vi "uut_status.vi"(8 "error in (no error)":errorcluster, 11 "status":bool) -> (0 "error out":errorcluster)   [LabVIEW 2019]
panel:
  out "String":string
  out "status":string
  # "UUT Status"
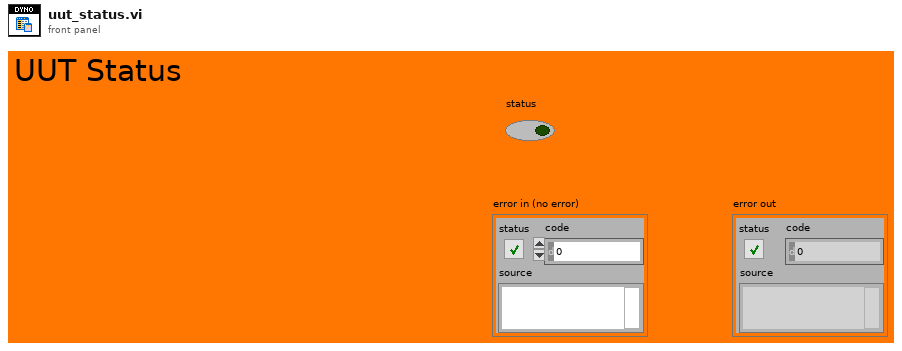
[diagram p1: front panel]
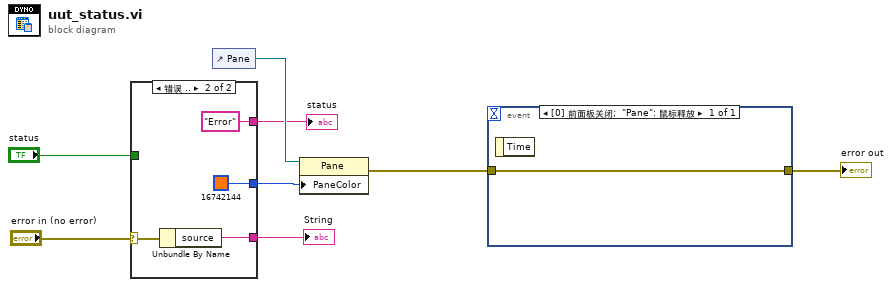
[diagram p0: block diagram]
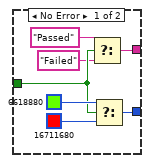
[diagram p2: hidden frame]
diagram:
  n1 = case shown="错误 .." "error in (no error)" {
    selector: "error in (no error)" -> [_ w17]
    tunnel: "status" -> [w12 _]
    tunnel: [w13 u32 16742144] -> w3
    tunnel: [w11 "Error"] -> w2
    tunnel: [_ w16] -> w1
    frame No Error {
      n2 = Select(t="Passed" ("status"), s=w12, f="Failed" ("status")) -> (s? t:f=w11:string)
      n3 = Select(t=u32 6618880, s=w12, f=u32 16711680) -> (s? t:f=w13:u32)
    }
    frame Error {
      n4 = Unbundle By Name(w17) -> ("source"=w16:string)
    }
  }
  "status" <- w2
  "String" <- w1
  n5 = control-ref of="Pane"() -> (w7:refnum<vi>)
  n6 = property class="Pane"(reference=w7, "PaneColor"=w3) -> (error out=w6:errorcluster)  [unwired: 1 in, 1 out]
  n7 = event shown="[0] 前面板关闭;  \"Pane\": 鼠标释放" {
    selector: _ -> [_]
    dyn-events: _ -> [_]
    timeout: _ -> [_]
    tunnel: [w20] -> w8
    tunnel: w6 -> [w20]
    event Panel Close; Mouse Up {
      n8 = event-data() -> ()  [unwired: 1 in, 1 out]
    }
  }
  "error out" <- w8
